vi "Asana Dictionary Get Value.vi"(8 "error in (no error)":errorcluster, 10 "Key":string, 11 "Data":T1(array[cluster])) -> (0 "error out":errorcluster, 3 "Value":string)   [LabVIEW 2016, in "Control Experiment.lvclass"]
uses:
  Control Experiment.lvclass
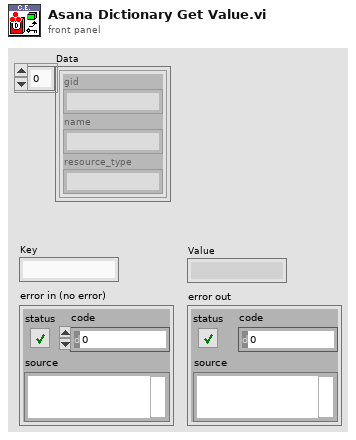
[diagram p1: front panel]
types:
  T1 = cluster{"gid":string, "name":string, "resource_type":string}[]
  T2 = typedef "Dictionary Object RefNum__ogtk.ctl" = refnum<k1>
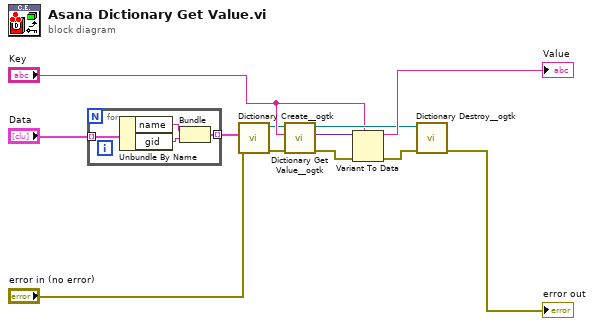
[diagram p0: block diagram]
diagram:
  n1 = for {
    tunnel: "Data" -> [w16] mode=indexing
    tunnel: [w13] -> w5 mode=indexing
    n2 = Unbundle By Name(w16) -> ("name"=w15:string, "gid"=w14:string)
    n3 = Bundle("name"=w15, "gid"=w14) -> (w13:cluster{"name":string, "gid":string})  [unwired: 1 in]
  }
  n4 = call <userlib>:"Dictionary Create__ogtk.vi"("error in (no error)"="error in (no error)", "initial dictionary (empty)"=w5) -> ("error out"=w2:errorcluster, "dictionary out"=w3:T2)  [unwired: 8 in]
  n5 = call <userlib>:"Dictionary Get Value__ogtk.vi"("error in"=w2, "key"="Key", "dictionary"=w3) -> ("error out"=w6:errorcluster, "value"=w7:variant, "dictionary out"=w10:T2)  [unwired: 5 in, 1 out]
  n6 = Variant To Data(error in=w6, type="Key", Variant=w7) -> (data=→"Value":string, error out=w9:errorcluster)
  n7 = call <userlib>:"Dictionary Destroy__ogtk.vi"("error in (no error)"=w9, "dictionary"=w10) -> ("error out"=→"error out":errorcluster)  [unwired: 9 in]
